vi "Right Click.vi"(7 "object refs":T2, 8 "error in (no error)":errorcluster, 9 "Coords":T1, 10 "Event data":variant, 11 "Data Grid in":refnum<class "Data Grid.lvclass">) -> (0 "error out":errorcluster, 3 "Data Grid out":refnum<class "Data Grid.lvclass">)   [LabVIEW 2013, in "Table Manager.lvlib" / "Data Grid.lvclass"]
uses:
  Data Grid.lvclass
  TagSelectModule/Source/editor node/object ref.ctl
  TagSelectModule/Source/editor node/tag select module editor node.lvclass
  <vilib>/NI/Tag Bus Data Framework/Configuration Editor/Classes/Engine Parent/Engine Parent Editor Node.lvclass
  <vilib>/Utility/miscctls.llb/LVPoint32TypeDef.ctl
  Table Manager/Table Manager.lvclass
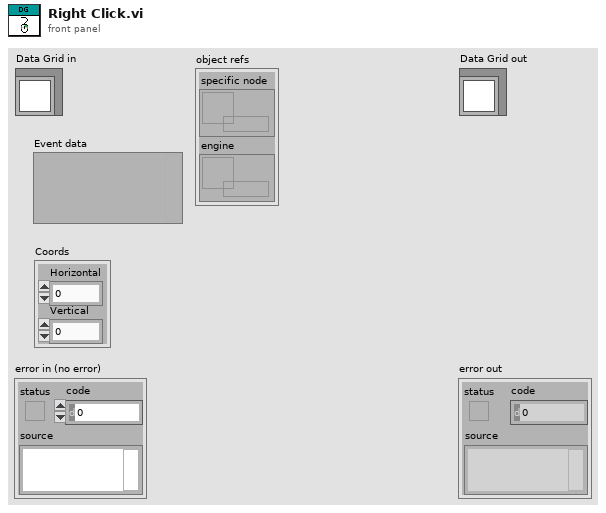
[diagram p1: front panel]
types:
  T1 = typedef "LVPoint32TypeDef.ctl" = cluster{"Horizontal":i32, "Vertical":i32}
  T2 = typedef "tag select module editor node.lvclass/object ref.ctl" = cluster{"specific node":refnum<data-value>, "engine":refnum<data-value>}
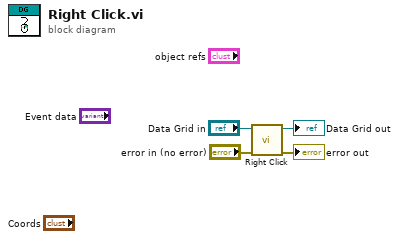
[diagram p0: block diagram]
diagram:
  n1 = call-parent "Right Click.vi"("error in (no error)"="error in (no error)", "Table Manager in"="Data Grid in") -> ("error out"=→"error out":errorcluster, "Table Manager out"=→"Data Grid out":refnum<class "Data Grid.lvclass">)  [unwired: 8 in]
